vi "DB Export Action - Export Parameters.vi"(8 "error in (no error)":errorcluster, 10 "selected path":path, 11 "Item Ref in":T9 format="%.0x") -> (0 "error out":errorcluster, 2 "selected path out":path caption="selected path", 3 "Item Ref out":T9 format="%.0x", 4 "Bus Out":T1)   [LabVIEW 2013, in "AIT 1553 Custom Device.lvlib"]
uses:
  AIT 1553 Custom Device.lvlib
  <vilib>/NI Veristand/Custom Device API/Custom Device Item Ref.ctl
  Controls/1553_Bus.ctl
  Controls/1553_Bus_Controller.ctl
  Controls/1553_BC_Message.ctl
  Controls/1553 Param.ctl
  Controls/1553_Acyclic_Frame.ctl
  Controls/1553_Bus_Monitor.ctl
  Controls/1553_BM_Message.ctl
  Controls/1553_RT_Message.ctl
  <vilib>/NI Veristand/Custom Device API/Custom Device API.lvlib
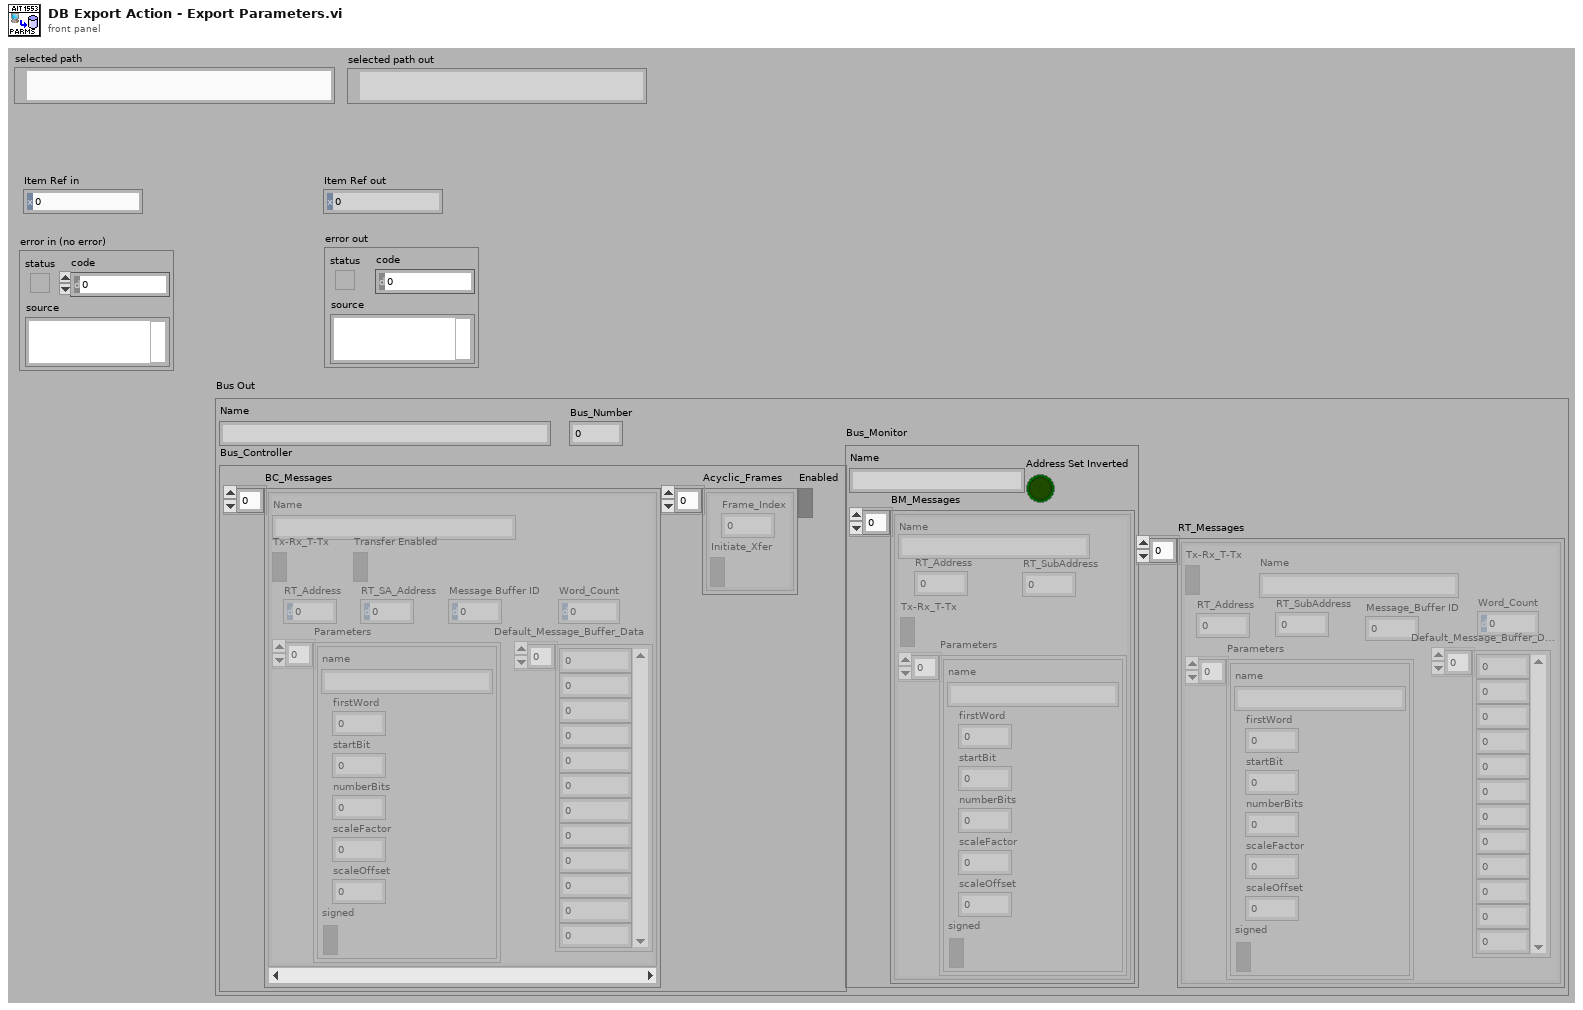
[diagram p1: front panel]
types:
  T1 = typedef "AIT 1553 Custom Device.lvlib/1553_Bus.ctl" = cluster{"Name":string, "Bus_Number":u8, "Bus_Controller":T2, "Bus_Monitor":T6, "RT_Messages":T8[]}
  T2 = typedef "AIT 1553 Custom Device.lvlib/1553_Bus_Controller.ctl" = cluster{"BC_Messages":T3[], "Acyclic_Frames":T5[], "Enabled":bool}
  T3 = typedef "AIT 1553 Custom Device.lvlib/1553_BC_Message.ctl" = cluster{"Name":string, "Tx-Rx_T-Tx":bool, "RT_Address":u8, "RT_SA_Address":u8, "Parameters":T4[], "Transfer Enabled":bool, "Message Buffer ID":u16, "Default_Message_Buffer_Data":u16[], "Word_Count":u8}
  T4 = typedef "AIT 1553 Custom Device.lvlib/1553 Param.ctl" = cluster{"name":string, "firstWord":i32, "startBit":i32, "numberBits":i32, "scaleFactor":dbl, "scaleOffset":dbl, "signed":bool}
  T5 = typedef "AIT 1553 Custom Device.lvlib/1553_Acyclic_Frame.ctl" = cluster{"Frame_Index":u8, "Initiate_Xfer":bool}
  T6 = typedef "AIT 1553 Custom Device.lvlib/1553_Bus_Monitor.ctl" = cluster{"Name":string, "BM_Messages":T7[], "Address Set Inverted":bool}
  T7 = typedef "AIT 1553 Custom Device.lvlib/1553_BM_Message.ctl" = cluster{"RT_Address":u8, "RT_SubAddress":u8, "Tx-Rx_T-Tx":bool, "Parameters":T4[], "Name":string}
  T8 = typedef "AIT 1553 Custom Device.lvlib/1553_RT_Message.ctl" = cluster{"RT_Address":u8, "RT_SubAddress":u8, "Tx-Rx_T-Tx":bool, "Parameters":T4[], "Message_Buffer ID":u16, "Default_Message_Buffer_Data":u16[], "Word_Count":u8, "Name":string}
  T9 = typedef "Custom Device API.lvlib/Custom Device Item Ref.ctl" = u64
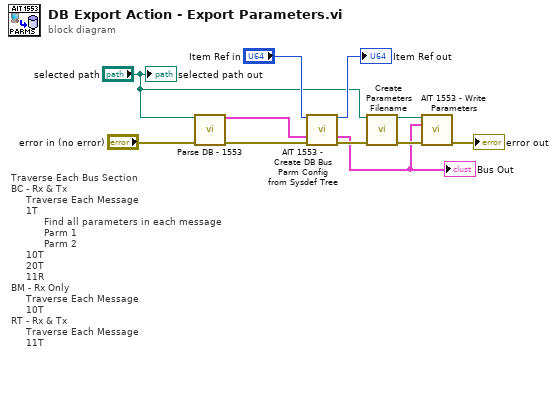
[diagram p0: block diagram]
diagram:
  # "Traverse Each Bus Section\nBC - Rx & Tx\n     Traverse Each Message\n     1T\n           Find all parameters in each message\n           Parm 1\n           Parm 2    \n     10T\n     20T\n     11R\nBM - Rx Only\n     Traverse Each Message\n     10T\nRT - Rx & Tx\n     Traverse Each Message\n     11T"
  n1 = call "Parse DB - 1553.vi"("Path in"="selected path", "error in (no error)"="error in (no error)") -> ("Bus"=w10:T1, "error out"=w8:errorcluster)  [unwired: 12 in]
  n2 = call "AIT 1553 - Create DB Bus Parm Config from Sysdef Tree.vi"("Device Ptr"="Item Ref in", "Bus"=w10, "error in"=w8) -> ("Device Ptr dup"=→"Item Ref out":u64, "Bus Out"=w1:T1, "error out"=w5:errorcluster)  [unwired: 10 in]
  "Bus Out" <- w1
  n3 = call "Create Parameters Filename.vi"("Simulyzer File Path"="selected path", "error in (no error)"=w5) -> ("Parm File Path"=w4:path, "error out"=w3:errorcluster)  [unwired: 12 in]
  n4 = call "AIT 1553 - Write Parameters.vi"("File Path"=w4, "Bus In"=w1, "error in (no error)"=w3) -> ("error out"=→"error out":errorcluster)  [unwired: 12 in]
  "selected path out" <- "selected path"
